vi "_Unpack for gRPC.vi"(8 "error in (no error)":errorcluster, 9 "Configuration / Resuls (Config)":enum16{"Configuration", "Results"}(ring), 10 "Any":T1, 11 "Measurement Customizations in":refnum<class "Measurement Plugin.lvclass">) -> (0 "error out":errorcluster, 2 "Data Value":variant, 3 "Measurement Customizations out":refnum<class "Measurement Plugin.lvclass">)   [LabVIEW 2020, in "VISA Measurement.lvlib" / "Measurement Plugin.lvclass"]
uses:
  Measurement Plugin.lvclass
  <vilib>/gRPC/LabVIEW gRPC Library/Shared/Any.ctl
  C:/Program Files/National Instruments/LabVIEW 2020/vi.lib/MeasurementLink/MeasurementLink Measurement Server/Measurement Plugin Service/Measurement Plugin Service.lvclass
  Measurement Configuration.ctl
  Measurement Results.ctl
  a521b266-ce99-437c-923d-067dcf1e07fd.vi
  3ecd018e-d556-4cbc-bc60-c4ba57204520.vi
  <vilib>/gRPC/LabVIEW gRPC Library/Server API/Translate Protobuf Error.vi
  <vilib>/AdvancedString/1D String Array to Delimited String.vi
  <vilib>/gRPC/LabVIEW gRPC Library/Server API/Server/Get Server DLL Path.vi
  VISA Measurement.lvlib
  <vilib>/MeasurementLink/MeasurementLink Measurement Server/Measurement Plugin Service/Measurement Plugin Service.lvclass
  <vilib>/gRPC/LabVIEW gRPC Library/grpc-lvsupport-release.lvlib
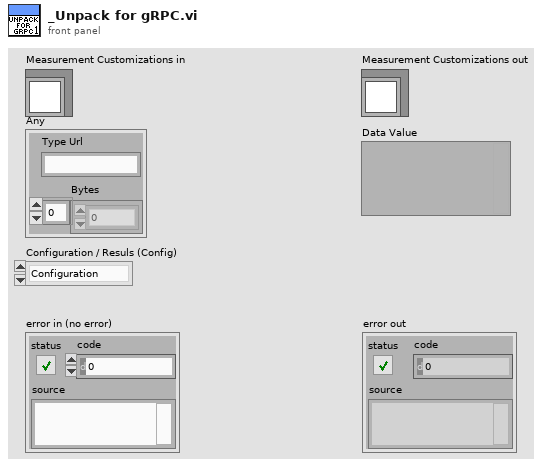
[diagram p1: front panel]
types:
  T1 = typedef "grpc-lvsupport-release.lvlib/Any.ctl" = cluster{"Type Url":string, "Bytes":u8[]}
  T2 = typedef "grpc-lvsupport-release.lvlib/grpcId.ctl" = u64
  T3 = typedef "VISA Measurement.lvlib/Measurement Configuration.ctl" = cluster{"pin name":string, "command":string, "baud rate":u32, "data bits":u32, "parity":enum32{"None", "Odd", "Even", "Mark", "Space"}, "stop bits":u32, "flow control":u32, "read byte count":u32, "end read on term char":bool, "end write on term char":bool}
  T4 = typedef "VISA Measurement.lvlib/Measurement Results.ctl" = cluster{"response":string}
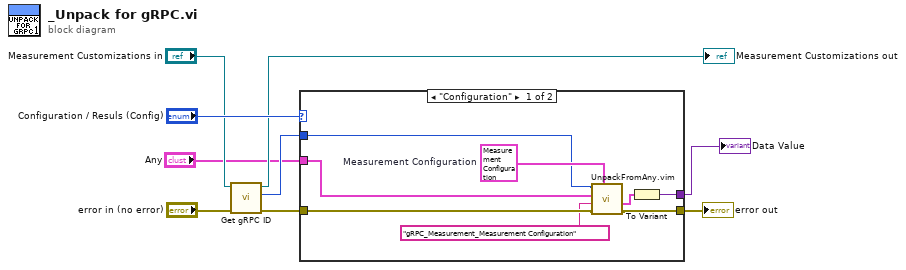
[diagram p0: block diagram]
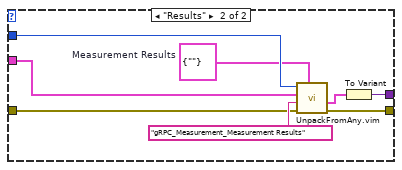
[diagram p2: hidden frame]
diagram:
  n1 = call <vilib>:"Get gRPC ID.vi"("error in (no error)"="error in (no error)", "MeasurementPluginService in"="Measurement Customizations in") -> ("error out"=w6:errorcluster, "gRPCid"=w3:T2, "MeasurementPluginService out"=→"Measurement Customizations out":refnum<class "Measurement Plugin.lvclass">)  [unwired: 7 in]
  n2 = case shown="\"Configuration\"" "Configuration / Resuls (Config)" {
    tunnel: w6 -> [w15 w19]
    tunnel: "Any" -> [w10 w18]
    tunnel: w3 -> [w12 w22]
    tunnel: [w16 w23] -> w9
    tunnel: [w17 w25] -> w1
    frame "Configuration" {
      w13 = T3 {"pin name"="", "command"="*IDN?", "baud rate"=9600, "data bits"=8, "parity"=enum."None", "stop bits"=0, "flow control"=0, "read byte count"=1000, "end read on term char"=TRUE, "end write on term char"=TRUE}  # Measurement Configuration
      n3 = call "UnpackFromAny.vim"("Data Type"=w13, "error in"=w15, "Message Type"="gRPC_Measurement_Measurement Configuration", "Any"=w10, "gRPCid in"=w12) -> ("error out"=w16:errorcluster, "Unpacked Value"=w14:T3)  [unwired: 4 in, 1 out]
      n4 = To Variant(anything=w14) -> (Variant=w17:variant)
    }
    frame "Results" {
      w21 = T4 {"response"=""}  # Measurement Results
      n5 = call "UnpackFromAny.vim"("Data Type"=w21, "error in"=w19, "Message Type"="gRPC_Measurement_Measurement Results", "Any"=w18, "gRPCid in"=w22) -> ("error out"=w23:errorcluster, "Unpacked Value"=w24:T4)  [unwired: 4 in, 1 out]
      n6 = To Variant(anything=w24) -> (Variant=w25:variant)
    }
  }
  "error out" <- w9
  "Data Value" <- w1
